vi "EL1002.vi"() -> ()   [LabVIEW 2022 SP3, in "IO_Library.lvlib"]
uses:
  IO_Library.lvlib
  ADS/ADS_Library.lvlib
  TypeDefs/EL1002Inputs.ctl
panel:
  out "EL1002 Inputs":T1
  in  "EL1002 Inputs":T1
  in  "error in (no error)":errorcluster
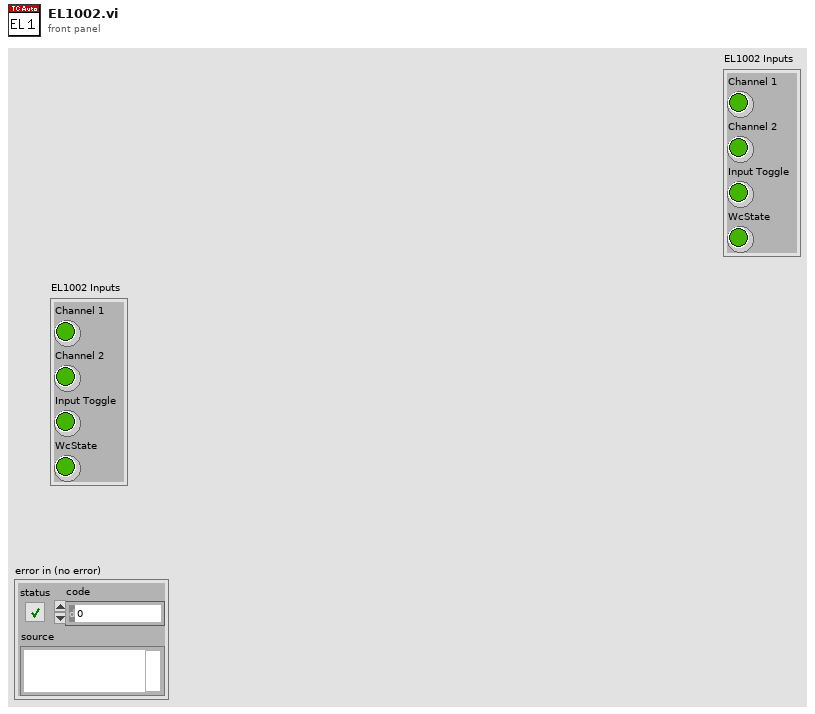
[diagram p1: front panel]
types:
  T1 = typedef "IO_Library.lvlib/EL1002Inputs.ctl" = cluster{"Channel 1":bool, "Channel 2":bool, "Input Toggle":bool, "WcState":bool}
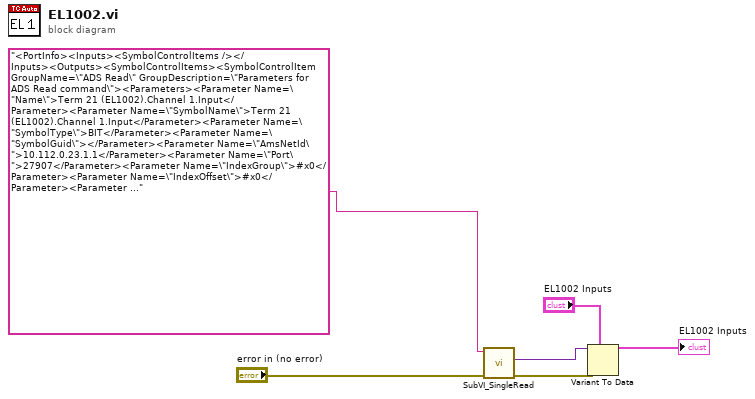
[diagram p0: block diagram]
diagram:
  n1 = call "SubVI_SingleRead.vi"("error in"="error in (no error)", "String"="<PortInfo><Inputs><SymbolControlItems /></Inputs><Outputs><SymbolControlItems><SymbolControlItem GroupName=\"ADS Read\" GroupDescription=\"Parameters for ADS Read command\"><Parameters><Parameter Name=\"Name\">Term 21 (EL1002).Channel 1.Input</Parameter><Parameter Name=\"SymbolName\">Term 21 (EL1002).Channel 1.Input</Parameter><Parameter Name=\"SymbolType\">BIT</Parameter><Parameter Name=\"SymbolGuid\"></Parameter><Parameter Name=\"AmsNetId\">10.112.0.23.1.1</Parameter><Parameter Name=\"Port\">27907</Parameter><Parameter Name=\"IndexGroup\">#x0</Parameter><Parameter Name=\"IndexOffset\">#x0</Parameter><Parameter Name=\"BitSize\">1</Parameter><Parameter Name=\"CycleTime [ms]\">10</Parameter><Parameter Name=\"Transmode\">3</Parameter><Parameter Name=\"Timeout [ms]\">1000</Parameter><Parameter Name=\"TCBufferSize [Samples]\">10</Parameter><Parameter Name=\"LVBufferSize [Samples]\">50</Parameter><Parameter Name=\"Expected min delay [ms]\">500</Parameter></Parameters></SymbolControlItem><SymbolControlItem GroupName=\"ADS Read\" GroupDescription=\"Parameters for ADS Read command\"><Parameters><Parameter Name=\"Name\">Term 21 (EL1002).Channel 2.Input</Parameter><Parameter Name=\"SymbolName\">Term 21 (EL1002).Channel 2.Input</Parameter><Parameter Name=\"SymbolType\">BIT</Parameter><Parameter Name=\"SymbolGuid\"></Parameter><Parameter Name=\"AmsNetId\">10.112.0.23.1.1</Parameter><Parameter Name=\"Port\">27907</Parameter><Parameter Name=\"IndexGroup\">#x0</Parameter><Parameter Name=\"IndexOffset\">#x0</Parameter><Parameter Name=\"BitSize\">1</Parameter><Parameter Name=\"CycleTime [ms]\">10</Parameter><Parameter Name=\"Transmode\">3</Parameter><Parameter Name=\"Timeout [ms]\">1000</Parameter><Parameter Name=\"TCBufferSize [Samples]\">10</Parameter><Parameter Name=\"LVBufferSize [Samples]\">50</Parameter><Parameter Name=\"Expected min delay [ms]\">500</Parameter></Parameters></SymbolControlItem><SymbolControlItem GroupName=\"ADS Read\" GroupDescription=\"Parameters for ADS Read command\"><Parameters><Parameter Name=\"Name\">Term 21 (EL1002).InputToggle</Parameter><Parameter Name=\"SymbolName\">Term 21 (EL1002).InputToggle</Parameter><Parameter Name=\"SymbolType\">BIT</Parameter><Parameter Name=\"SymbolGuid\"></Parameter><Parameter Name=\"AmsNetId\">10.112.0.23.1.1</Parameter><Parameter Name=\"Port\">27907</Parameter><Parameter Name=\"IndexGroup\">#x0</Parameter><Parameter Name=\"IndexOffset\">#x0</Parameter><Parameter Name=\"BitSize\">1</Parameter><Parameter Name=\"CycleTime [ms]\">10</Parameter><Parameter Name=\"Transmode\">3</Parameter><Parameter Name=\"Timeout [ms]\">1000</Parameter><Parameter Name=\"TCBufferSize [Samples]\">10</Parameter><Parameter Name=\"LVBufferSize [Samples]\">50</Parameter><Parameter Name=\"Expected min delay [ms]\">500</Parameter></Parameters></SymbolControlItem><SymbolControlItem GroupName=\"ADS Read\" GroupDescription=\"Parameters for ADS Read command\"><Parameters><Parameter Name=\"Name\">Term 21 (EL1002).WcState</Parameter><Parameter Name=\"SymbolName\">Term 21 (EL1002).WcState</Parameter><Parameter Name=\"SymbolType\">BIT</Parameter><Parameter Name=\"SymbolGuid\"></Parameter><Parameter Name=\"AmsNetId\">10.112.0.23.1.1</Parameter><Parameter Name=\"Port\">27907</Parameter><Parameter Name=\"IndexGroup\">#x0</Parameter><Parameter Name=\"IndexOffset\">#x0</Parameter><Parameter Name=\"BitSize\">1</Parameter><Parameter Name=\"CycleTime [ms]\">10</Parameter><Parameter Name=\"Transmode\">3</Parameter><Parameter Name=\"Timeout [ms]\">1000</Parameter><Parameter Name=\"TCBufferSize [Samples]\">10</Parameter><Parameter Name=\"LVBufferSize [Samples]\">50</Parameter><Parameter Name=\"Expected min delay [ms]\">500</Parameter></Parameters></SymbolControlItem></SymbolControlItems></Outputs></PortInfo>") -> ("error out"=w3:errorcluster, "RData"=w4:variant)  [unwired: 6 in, 1 out]
  n2 = Variant To Data(error in=w3, type="EL1002 Inputs", Variant=w4) -> (data=→"EL1002 Inputs":T1)  [unwired: 1 out]
